vi "MyTestClass_Create.vi"(0 "reference in":refnum<class "MyTestClass.lvclass">, 5 "error in (no error)":errorcluster) -> (14 "reference out":refnum<class "MyTestClass.lvclass">, 19 "error out":errorcluster)   [LabVIEW 2020, in "MyTestClass.lvclass"]
doc: "Constructor."
uses:
  MyTestClass.lvclass
  C:/ProjectGSharpDevelopment_2020-3/gsharp/VIPM/Files/vi.lib/addons/_AddQ/G#Object/G#Object.lvclass
  vi.lib/addons/_AddQ/G#Object/G#Object.lvclass
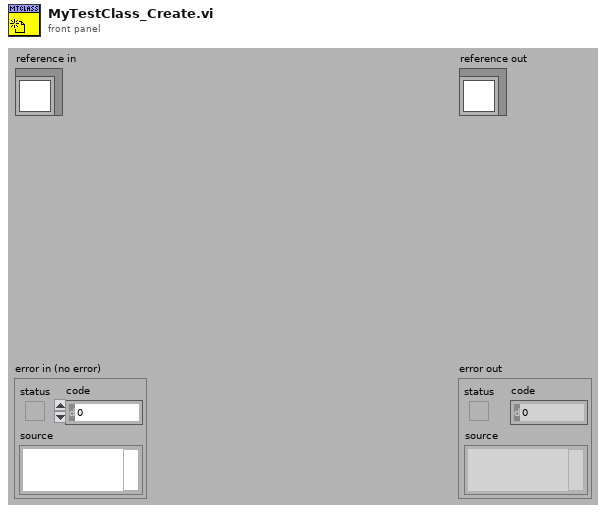
[diagram p1: front panel]
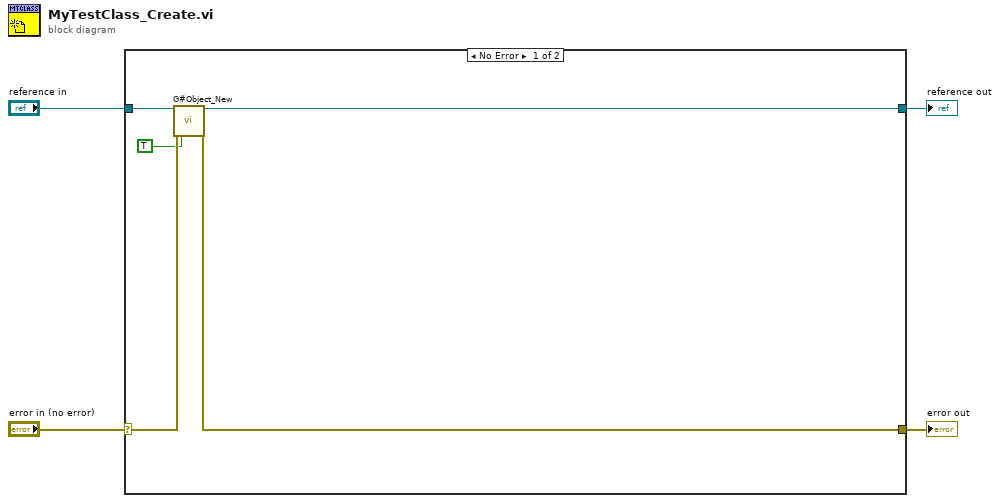
[diagram p0: block diagram]
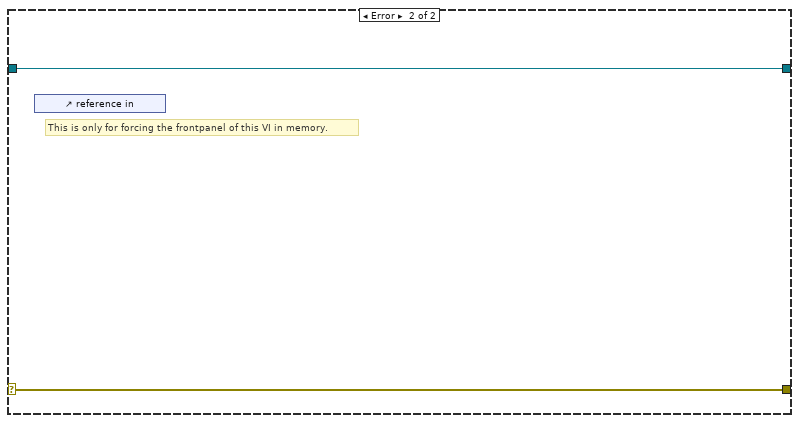
[diagram p2: hidden frame]
diagram:
  n1 = case shown="No Error" "error in (no error)" {
    selector: "error in (no error)" -> [w8 w11]
    tunnel: [w5 w11] -> w3
    tunnel: [w6 w10] -> w1
    tunnel: "reference in" -> [w9 w10]
    frame No Error {
      n2 = call "G#Object_New.vi"("reference in"=w9, "error in (no error)"=w8, "user counter (T)?"=TRUE ("User Counter")) -> ("reference out"=w6:refnum<class "MyTestClass.lvclass">, "error out"=w5:errorcluster)  [unwired: 14 in, 1 out]
    }
    frame Error {
      # "This is only for forcing the frontpanel of this VI in memory."
      n3 = control-ref of="reference in"() -> ()  [unwired: 1 out]
    }
  }
  "error out" <- w3
  "reference out" <- w1
